vi "Get Instrument Type ID.vi"(8 "error in":errorcluster, 11 "instrument in":refnum<class "Fake Instrument.lvclass">) -> (0 "error out":errorcluster, 2 "instrument type id":string, 3 "instrument out":refnum<class "Fake Instrument.lvclass">)   [LabVIEW 2020, in "MeasurementServerTests.lvlib" / "Fake Instrument.lvclass"]
uses:
  Fake Instrument.lvclass
  Fake Instrument.lvclass/Fake Instrument.ctl
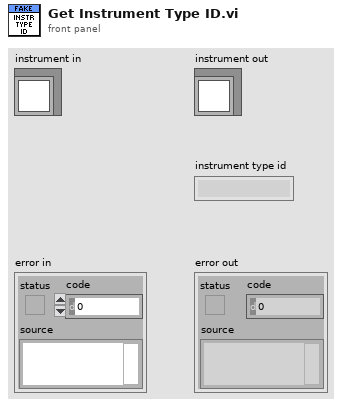
[diagram p1: front panel]
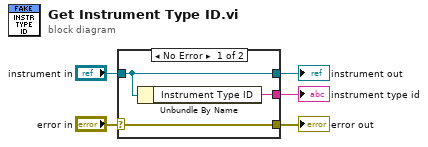
[diagram p0: block diagram]
diagram:
  n1 = case shown="No Error" "error in" {
    selector: "error in" -> [w7 w10]
    tunnel: "instrument in" -> [w6 w9]
    tunnel: [w8 _] -> w4
    tunnel: [w7 w10] -> w2
    tunnel: [w6 w9] -> w1
    frame No Error {
      n2 = Unbundle By Name(w6) -> ("Instrument Type ID"=w8:string)
    }
    frame Error {
    }
  }
  "error out" <- w2
  "instrument type id" <- w4
  "instrument out" <- w1
